vi "CheckFolder.vi"(8 "Overwrite?":bool, 9 "Index":u32, 10 "File Name":string, 11 "Folder Path Control":path) -> (1 "Warning":bool, 2 "Message":string, 3 "File Path":path)   [LabVIEW 2014]
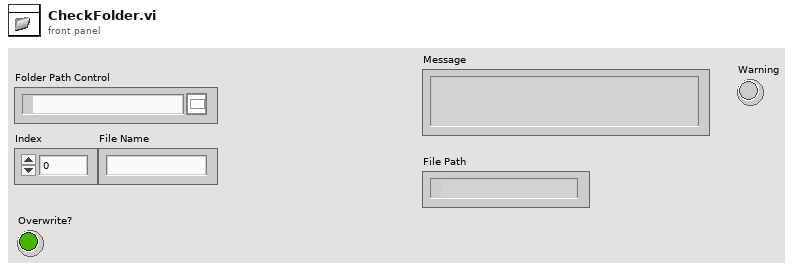
[diagram p1: front panel]
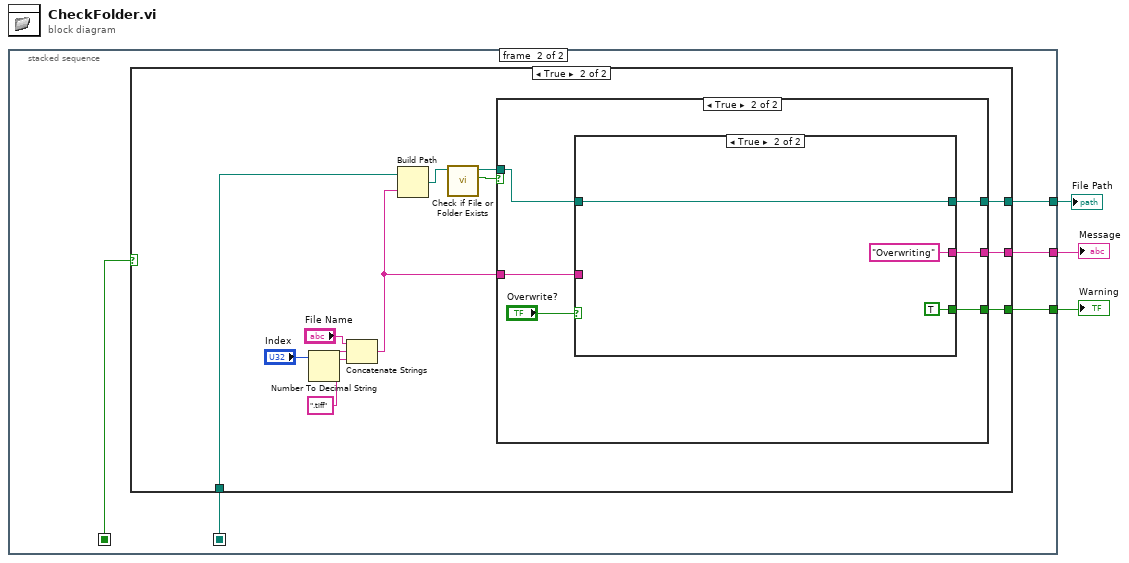
[diagram p0: block diagram]
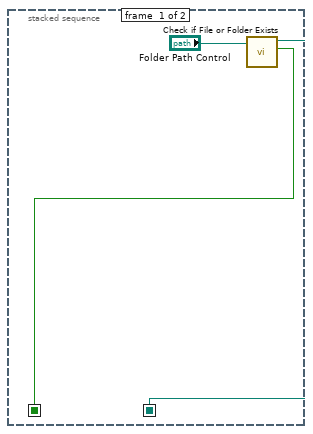
[diagram p2: hidden frame]
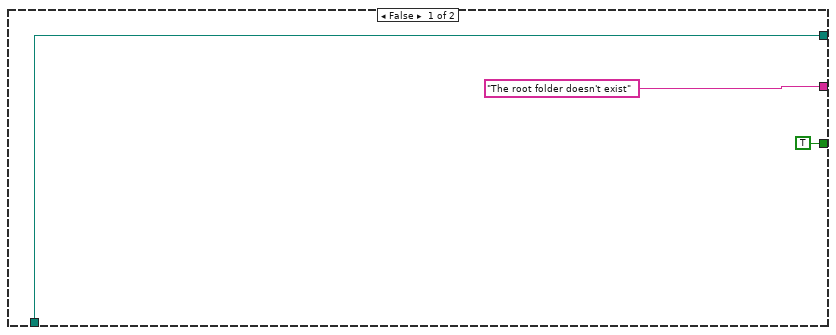
[diagram p3: hidden frame]
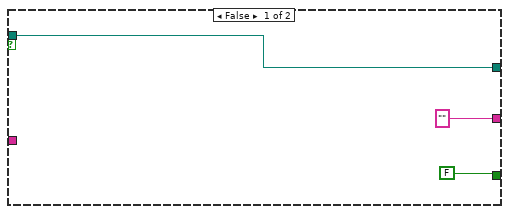
[diagram p4: hidden frame]
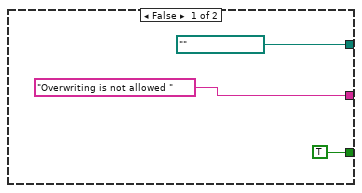
[diagram p5: hidden frame]
diagram:
  n1 = stacked-sequence {
    seq-local: [w5 _] -> [_ w7]
    seq-local: [w4 _] -> [_ w8]
    tunnel: [_ w11] -> w3
    tunnel: [_ w10] -> w2
    tunnel: [_ w9] -> w1
    frame #0 {
      n2 = call <vilib>:"Check if File or Folder Exists.vi"("path"="Folder Path Control") -> ("file or folder exists?"=w4:bool, "dup path"=w5:path)  [unwired: 8 in, 1 out]
    }
    frame #1 {
      n3 = case shown="True" w8 {
        tunnel: w7 -> [w14 w22]
        tunnel: [w14 w20] -> w11
        tunnel: [TRUE w19] -> w10
        tunnel: ["The root folder doesn't exist" w16] -> w9
        frame False {
        }
        frame True {
          n4 = Number To Decimal String(number="Index") -> (decimal integer string=w24:string)  [unwired: 1 in]
          n5 = Concatenate Strings("File Name", w24, ".tiff" ("string")) -> (w15:string)
          n6 = Build Path(base path=w22, name or relative path=w15) -> (appended path=w21:path)
          n7 = call <vilib>:"Check if File or Folder Exists.vi"("path"=w21) -> ("file or folder exists?"=w17:bool, "dup path"=w18:path)  [unwired: 8 in, 1 out]
          n8 = case shown="True" w17 {
            tunnel: [w29 w35] -> w20
            tunnel: [FALSE w34] -> w19
            tunnel: w18 -> [w29 w32]
            tunnel: ["" ("Message") w31] -> w16
            tunnel: w15 -> [_ w30]
            frame False {
            }
            frame True {
              n9 = case shown="True" "Overwrite?" {
                tunnel: [path "" ("File Path") w41] -> w35
                tunnel: [TRUE TRUE] -> w34
                tunnel: w32 -> [_ w41]
                tunnel: ["Overwriting is not allowed " ("Message") "Overwriting" ("Message")] -> w31
                tunnel: w30 -> [_ _]
                frame False {
                }
                frame True {
                }
              }
            }
          }
        }
      }
    }
  }
  "File Path" <- w3
  "Warning" <- w2
  "Message" <- w1
